vi "Set pressure auto-adjust.vi"(8 "error in (no error)":errorcluster, 9 "Target pressure range":T1, 10 "Enable?":bool, 11 "Pressure Control in":refnum<class "Pressure Control.lvclass">) -> (0 "error out":errorcluster, 3 "Pressure Control out":refnum<class "Pressure Control.lvclass">)   [LabVIEW 2011, in "Pressure Control.lvclass"]
uses:
  Pressure Control.lvclass
  Auto-adjust Pressure Range.ctl
  COSYLib/COSYLib.lvlib
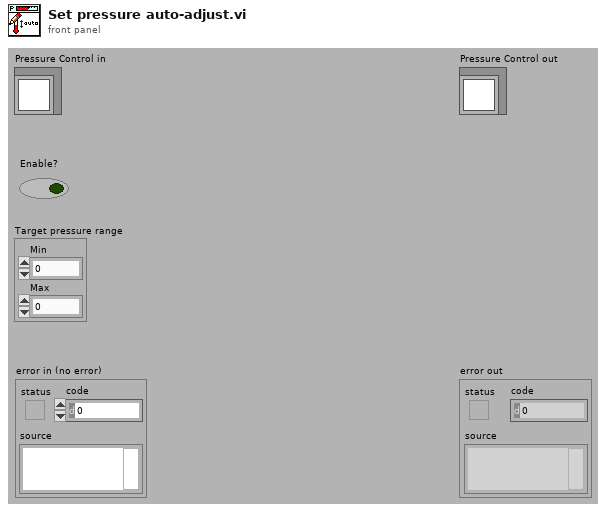
[diagram p1: front panel]
types:
  T1 = typedef "Pressure Control.lvclass/Auto-adjust Pressure Range.ctl" = cluster{"Min":dbl, "Max":dbl}
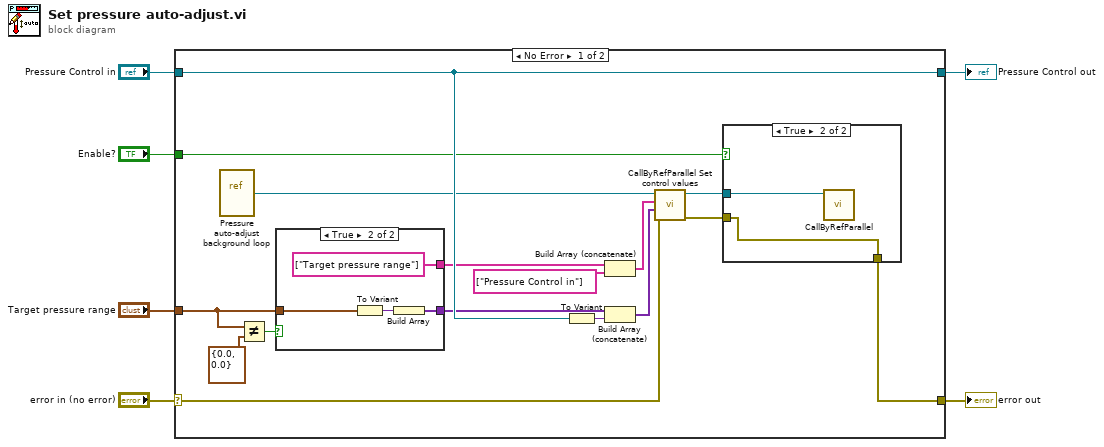
[diagram p0: block diagram]
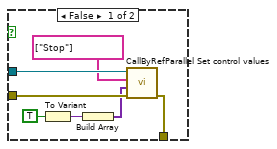
[diagram p2: hidden frame]
diagram:
  n1 = case shown="No Error" "error in (no error)" {
    selector: "error in (no error)" -> [w20 w37]
    tunnel: "Pressure Control in" -> [w22 w36]
    tunnel: "Enable?" -> [w7 _]
    tunnel: "Target pressure range" -> [w21 _]
    tunnel: [w22 w36] -> w1
    tunnel: [w18 w37] -> w2
    frame No Error {
      n2 = vi-ref "Pressure auto-adjust background loop.vi"() -> (w19:refnum<vi>)
      n3 = Not Equal?(x=w21, y=T1 {"Min"=0.0, "Max"=0.0}) -> (x != y?=w16:bool)
      n4 = case shown="True" w16 {
        tunnel: [_ string[] ["Target pressure range"]] -> w15
        tunnel: w21 -> [_ w34]
        tunnel: [_ w32] -> w13
        frame False {
        }
        frame True {
          n5 = To Variant(anything=w34) -> (Variant=w33:variant)
          n6 = Build Array(w33) -> (w32:variant[])
        }
      }
      n7 = To Variant(anything=w22) -> (Variant=w12:variant)
      n8 = Build Array (concatenate)(w15, string[] ["Pressure Control in"] ("array")) -> (w9:string[])
      n9 = Build Array (concatenate)(w13, w12) -> (w8:variant[])
      n10 = call "CallByRefParallel Set control values.vi"("error in (no error)"=w20, "Control values"=w8, "Control names"=w9, "VI Refnum"=w19) -> ("error out"=w10:errorcluster, "VI Refnum dup"=w11:refnum<vi>)  [unwired: 6 in]
      n11 = case shown="True" w7 {
        tunnel: [w26 w30] -> w18
        tunnel: w11 -> [w29 w31]
        tunnel: w10 -> [w28 w30]
        frame False {
          n12 = To Variant(anything=TRUE) -> (Variant=w24:variant)
          n13 = Build Array(w24) -> (w23:variant[])
          n14 = call "CallByRefParallel Set control values.vi"("error in (no error)"=w28, "Control values"=w23, "Control names"=string[] ["Stop"], "VI Refnum"=w29) -> ("error out"=w26:errorcluster)  [unwired: 6 in, 1 out]
        }
        frame True {
          n15 = call "CallByRefParallel.vi"("VI Refnum"=w31) -> ()  [unwired: 9 in, 2 out]
        }
      }
    }
    frame Error {
    }
  }
  "error out" <- w2
  "Pressure Control out" <- w1
